vi "Build Start Stop Graph Legend.vi"() -> (2 "Stop Legend Graph":string, 3 "Start Legend Graph":string)   [LabVIEW 2021, in "TAF Proj Document Type.lvlib" / "TAF Proj.lvclass"]
uses:
  <vilib>/Wovalab/AntiDoc/Document Type/Add-ons/LabVIEW TAF Project/TAF Proj/TAF Proj.lvclass
  <vilib>/Wovalab/AntiDoc/GraphBuilder/Renderer/Graphviz/Graphviz.lvclass
  C:/Program Files (x86)/National Instruments/LabVIEW 2021/vi.lib/Wovalab/AntiDoc/GraphBuilder/Renderer/Renderer.lvclass
  <vilib>/Wovalab/AntiDoc/GraphBuilder/Shapes/Edge/Graphviz/Graphviz Edge Shape.lvclass
  <vilib>/Wovalab/AntiDoc/GraphBuilder/Shapes/Edge/Graphviz/Shape.ctl
  <vilib>/Wovalab/AntiDoc/GraphBuilder/Shapes/Edge/Graphviz/Colors.ctl
  <vilib>/Wovalab/AntiDoc/GraphBuilder/Shapes/Node/Graphviz/Colors.ctl
  <vilib>/Wovalab/AntiDoc/GraphBuilder/Shapes/Node/Graphviz/Shape.ctl
  <vilib>/Wovalab/AntiDoc/GraphBuilder/Renderer/Graphviz/Graph Direction.ctl
  <vilib>/Wovalab/AntiDoc/GraphBuilder/Renderer/Graphviz/Specific Edge Shape Def.ctl
  <vilib>/Wovalab/AntiDoc/GraphBuilder/Renderer/Graphviz/Specific Node Shape Def.ctl
  <vilib>/Wovalab/AntiDoc/GraphBuilder/Shapes/Node/Graphviz/Graphviz Node Shape.lvclass
  <vilib>/Wovalab/AntiDoc/GraphBuilder/Node/Node.lvclass
  <vilib>/Wovalab/AntiDoc/GraphBuilder/Graph/Graph.lvclass
  <vilib>/Wovalab/AntiDoc/GraphBuilder/Edge/Edge.lvclass
  <vilib>/Wovalab/AntiDoc/Document Type/Add-ons/LabVIEW TAF Project/TAF Proj Document Type.lvlib
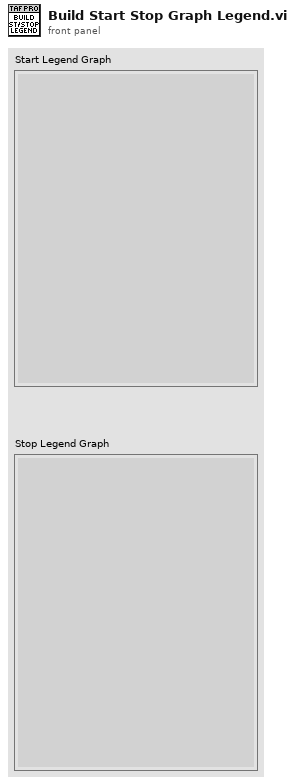
[diagram p1: front panel]
types:
  T1 = typedef "GraphBuilder.lvlib/Graphviz Edge Shape.lvclass/Shape.ctl" = enum16{"box", "lbox", "rbox", "obox", "olbox", "orbox", "crow", "lcrow", "rcrow", "diamond", "ldiamond", "rdiamond", "odiamond", "oldiamond", "ordiamond", "dot", "odot", "inv", "linv", "rinv", "oinv", "olinv", "orinv", "none", "normal", "lnormal", "rnormal", "onormal", "olnormal", "ornormal", "tee", "ltee", "rtee", "vee", "lvee", "rvee", "curve", "lcurve", "rcurve", "icurve", "licurve", "ricurve"}
  T2 = typedef "GraphBuilder.lvlib/Graphviz Edge Shape.lvclass/Style.ctl" = enum8{"filled", "invisible", "diagonals", "rounded", "dashed", "dotted", "solid", "bold"}
  T3 = typedef "GraphBuilder.lvlib/Graphviz Edge Shape.lvclass/Colors.ctl" = enum16{"aliceblue", "antiquewhite", "aqua", "aquamarine", "azure", "beige", "bisque", "black", "blanchedalmond", "blue", "blueviolet", "brown", "burlywood", "cadetblue", "chartreuse", "chocolate", "coral", "cornflowerblue", "cornsilk", "crimson", "cyan", "darkblue", "darkcyan", "darkgoldenrod", "darkgray", "darkgreen", "darkgrey", "darkkhaki", "darkmagenta", "darkolivegreen", "darkorange", "darkorchid", "darkred", "darksalmon", "darkseagreen", "darkslateblue", "darkslategray", "darkslategrey", "darkturquoise", "darkviolet", "deeppink", "deepskyblue", "dimgray", "dimgrey", "dodgerblue", "firebrick", "floralwhite", "forestgreen", "fuchsia", "gainsboro", "ghostwhite", "gold", "goldenrod", "gray", "green", "greenyellow", "grey", "honeydew", "hotpink", "indianred", "indigo", "ivory", "khaki", "lavender", "lavenderblush", "lawngreen", "lemonchiffon", "lightblue", "lightcoral", "lightcyan", "lightgoldenrodyellow", "lightgray", "lightgreen", "lightgrey", "lightpink", "lightsalmon", "lightseagreen", "lightskyblue", "lightslategray", "lightslategrey", "lightsteelblue", "lightyellow", "lime", "limegreen", "linen", "magenta", "maroon", "mediumaquamarine", "mediumblue", "mediumorchid", "mediumpurple", "mediumseagreen", "mediumslateblue", "mediumspringgreen", "mediumturquoise", "mediumvioletred", "midnightblue", "mintcream", "mistyrose", "moccasin", "navajowhite", "navy", "oldlace", "olive", "olivedrab", "orange", "orangered", "orchid", "palegoldenrod", "palegreen", "paleturquoise", "palevioletred", "papayawhip", "peachpuff", "peru", "pink", "plum", "powderblue", "purple", "red", "rosybrown", "royalblue", "saddlebrown", "salmon", "sandybrown", "seagreen", "seashell", "sienna", "silver", "skyblue", "slateblue", "slategray", "slategrey", "snow", "springgreen", "steelblue", "tan", "teal", "thistle", "tomato", "turquoise", "violet", "wheat", "white", "whitesmoke", "yellow", "yellowgreen"}
  T4 = typedef "GraphBuilder.lvlib/Graphviz Node Shape.lvclass/Colors.ctl" = enum16{"aliceblue", "antiquewhite", "aqua", "aquamarine", "azure", "beige", "bisque", "black", "blanchedalmond", "blue", "blueviolet", "brown", "burlywood", "cadetblue", "chartreuse", "chocolate", "coral", "cornflowerblue", "cornsilk", "crimson", "cyan", "darkblue", "darkcyan", "darkgoldenrod", "darkgray", "darkgreen", "darkgrey", "darkkhaki", "darkmagenta", "darkolivegreen", "darkorange", "darkorchid", "darkred", "darksalmon", "darkseagreen", "darkslateblue", "darkslategray", "darkslategrey", "darkturquoise", "darkviolet", "deeppink", "deepskyblue", "dimgray", "dimgrey", "dodgerblue", "firebrick", "floralwhite", "forestgreen", "fuchsia", "gainsboro", "ghostwhite", "gold", "goldenrod", "gray", "green", "greenyellow", "grey", "honeydew", "hotpink", "indianred", "indigo", "ivory", "khaki", "lavender", "lavenderblush", "lawngreen", "lemonchiffon", "lightblue", "lightcoral", "lightcyan", "lightgoldenrodyellow", "lightgray", "lightgreen", "lightgrey", "lightpink", "lightsalmon", "lightseagreen", "lightskyblue", "lightslategray", "lightslategrey", "lightsteelblue", "lightyellow", "lime", "limegreen", "linen", "magenta", "maroon", "mediumaquamarine", "mediumblue", "mediumorchid", "mediumpurple", "mediumseagreen", "mediumslateblue", "mediumspringgreen", "mediumturquoise", "mediumvioletred", "midnightblue", "mintcream", "mistyrose", "moccasin", "navajowhite", "navy", "oldlace", "olive", "olivedrab", "orange", "orangered", "orchid", "palegoldenrod", "palegreen", "paleturquoise", "palevioletred", "papayawhip", "peachpuff", "peru", "pink", "plum", "powderblue", "purple", "red", "rosybrown", "royalblue", "saddlebrown", "salmon", "sandybrown", "seagreen", "seashell", "sienna", "silver", "skyblue", "slateblue", "slategray", "slategrey", "snow", "springgreen", "steelblue", "tan", "teal", "thistle", "tomato", "turquoise", "violet", "wheat", "white", "whitesmoke", "yellow", "yellowgreen"}
  T5 = typedef "GraphBuilder.lvlib/Graphviz Node Shape.lvclass/Shape.ctl" = enum16{"box", "polygon", "ellipse", "oval", "circle", "point", "egg", "triangle", "plaintext", "plain", "diamond", "trapezium", "parallelogram", "house", "pentagon", "hexagon", "septagon", "octagon", "doublecircle", "doubleoctagon", "tripleoctagon", "invtriangle", "invtrapezium", "invhouse", "Mdiamond", "Msquare", "Mcircle", "rect", "rectangle", "square", "star", "none", "underline", "cylinder", "note", "tab", "folder", "box3D", "component", "promoter", "cds", "terminator", "utr", "primersite", "restrictionsite", "fivepoverhang", "threepoverhang", "noverhang", "assembly", "signature", "insulator", "ribosite", "rnastab", "proteasesite", "proteinstab", "rpromoter", "rarrow", "larrow", "lpromoter"}
  T6 = typedef "GraphBuilder.lvlib/Graphviz.lvclass/Specific Node Shape Def.ctl" = cluster{"Node ID":string, "Graphviz Node Shape":refnum<class "Graphviz Node Shape.lvclass">}
  T7 = typedef "GraphBuilder.lvlib/Graphviz.lvclass/Specific Edge Shape Def.ctl" = cluster{"Source Node ID":string, "Target Node ID":string, "Caption":string, "Graphviz Edge Shape":refnum<class "Graphviz Edge Shape.lvclass">}
  T8 = typedef "GraphBuilder.lvlib/Graphviz.lvclass/Graph Direction.ctl" = enum16{"Top to Bottom", "Left To Right", "Bottom to Top", "Right to Left"}
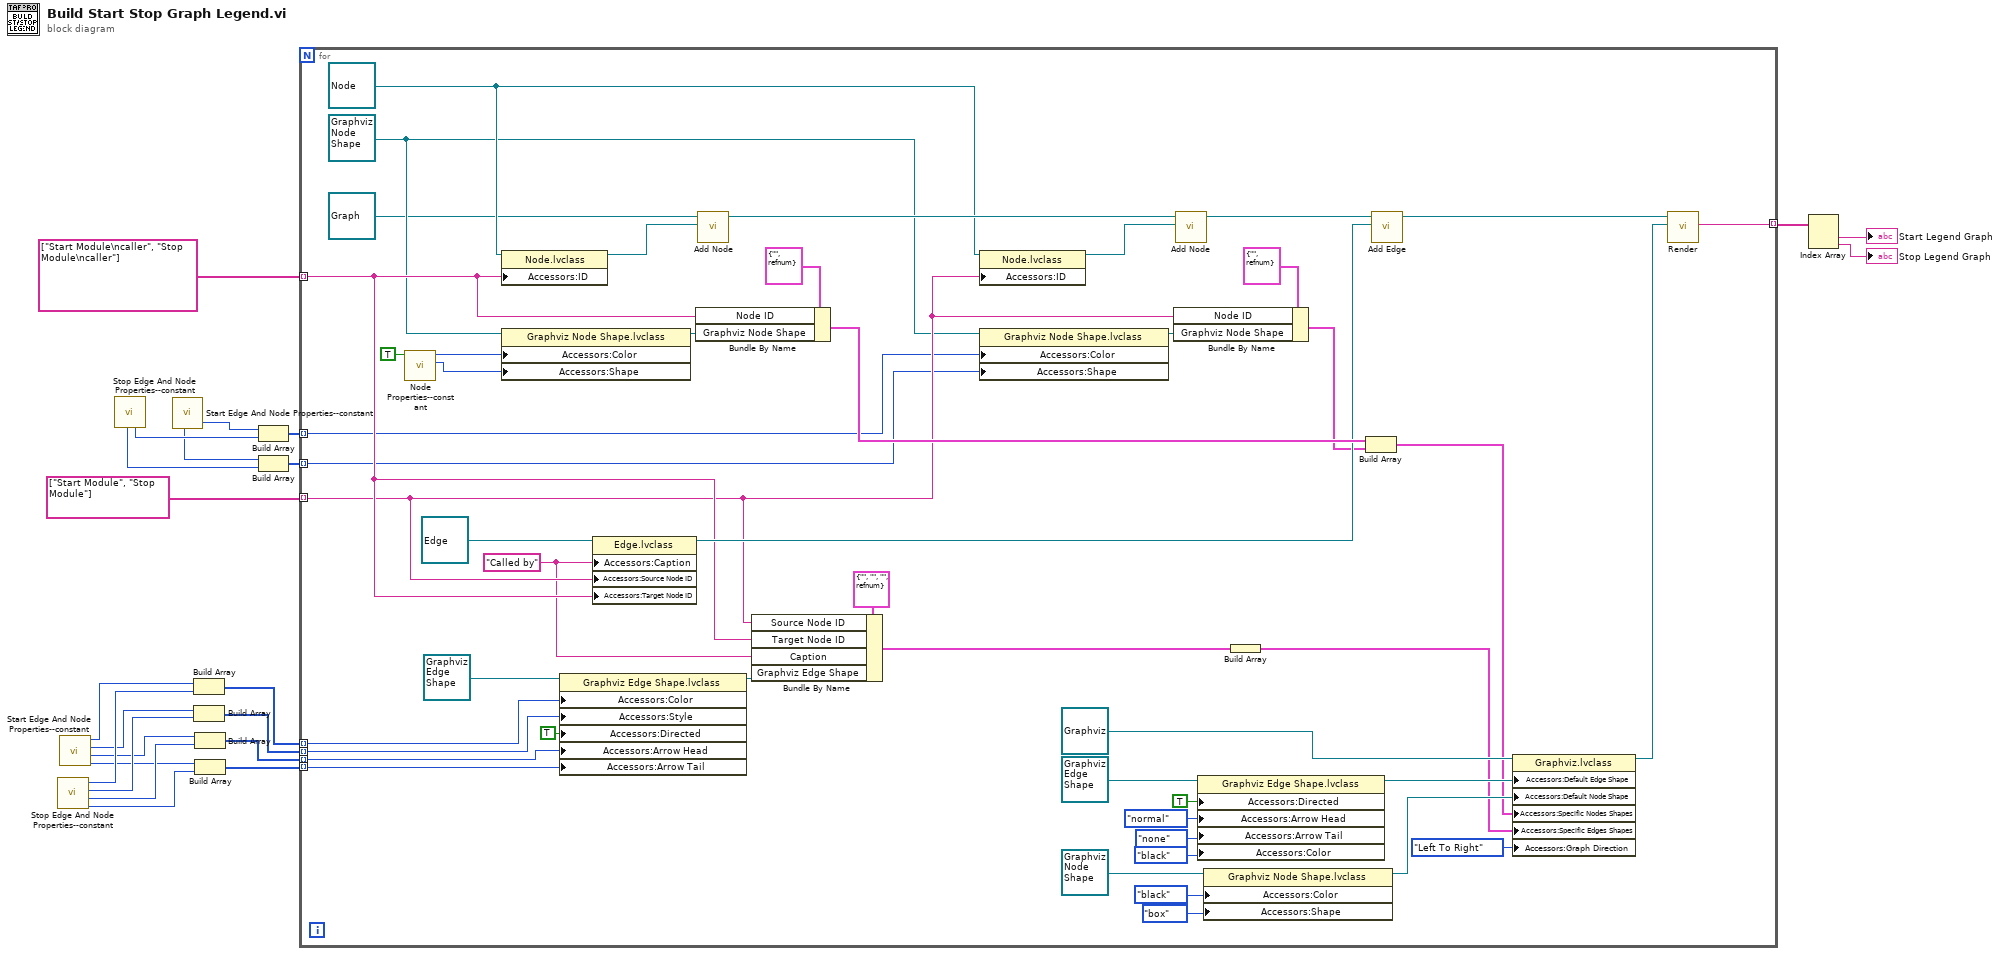
[diagram p0: block diagram]
diagram:
  n1 = call <vilib>:"Stop Edge And Node Properties--constant.vi"() -> ("Edge Arrow Tail"=w12:T1, "Edge Arrow Head"=w13:T1, "Edge Style"=w14:T2, "Edge Color"=w15:T3)  [unwired: 6 in, 2 out]
  n2 = call <vilib>:"Start Edge And Node Properties--constant.vi"() -> ("Edge Arrow Tail"=w5:T1, "Edge Arrow Head"=w7:T1, "Edge Style"=w9:T2, "Edge Color"=w11:T3)  [unwired: 6 in, 2 out]
  n3 = call <vilib>:"Stop Edge And Node Properties--constant.vi"() -> ("Node Color"=w20:T4, "Node Shape"=w18:T5)  [unwired: 6 in, 4 out]
  n4 = call <vilib>:"Start Edge And Node Properties--constant.vi"() -> ("Node Color"=w21:T4, "Node Shape"=w19:T5)  [unwired: 6 in, 4 out]
  n5 = Build Array(w11, w15) -> (w10:T3[])
  n6 = Build Array(w9, w14) -> (w8:T2[])
  n7 = Build Array(w7, w13) -> (w6:T1[])
  n8 = Build Array(w5, w12) -> (w4:T1[])
  n9 = Build Array(w21, w20) -> (w17:T4[])
  n10 = Build Array(w19, w18) -> (w16:T5[])
  n11 = for {
    tunnel: [w54] -> w3 mode=indexing
    tunnel: string[] ["Start Module\ncaller", "Stop Module\ncaller"] -> [w47] mode=indexing
    tunnel: w10 -> [w46] mode=indexing
    tunnel: w8 -> [w45] mode=indexing
    tunnel: w6 -> [w44] mode=indexing
    tunnel: w4 -> [w43] mode=indexing
    tunnel: string[] ["Start Module", "Stop Module"] -> [w38] mode=indexing
    tunnel: w17 -> [w34] mode=indexing
    tunnel: w16 -> [w33] mode=indexing
    w24 = "Called by" ("Caption")
    w28 = refnum<class "Graphviz Node Shape.lvclass"> refnum ("GraphBuilder.lvlib:Graphviz Node Shape.lvclass")
    w29 = refnum<class "Node.lvclass"> refnum ("GraphBuilder.lvlib:Node.lvclass")
    n12 = call <vilib>:"Node Properties--constant.vi"("Lvlib"=TRUE) -> ("Shape"=w49:T5, "Color"=w50:T4)  [unwired: 9 in]
    n13 = property class="Node.lvclass"(reference=w29, "Accessors:ID"=w47) -> (reference out=w30:refnum<class "Node.lvclass">)  [unwired: 1 in, 1 out]
    n14 = property class="Graphviz Node Shape.lvclass"(reference=w28, "Accessors:Color"=w50, "Accessors:Shape"=w49) -> (reference out=w32:refnum<class "Graphviz Node Shape.lvclass">)  [unwired: 1 in, 1 out]
    n15 = property class="Graphviz Edge Shape.lvclass"(reference=refnum<class "Graphviz Edge Shape.lvclass"> refnum ("Graphviz Edge Shape"), "Accessors:Color"=w46, "Accessors:Style"=w45, "Accessors:Directed"=TRUE ("Directed"), "Accessors:Arrow Head"=w44, "Accessors:Arrow Tail"=w43) -> (reference out=w59:refnum<class "Graphviz Edge Shape.lvclass">)  [unwired: 1 in, 1 out]
    n16 = property class="Edge.lvclass"(reference=refnum<class "Edge.lvclass"> refnum ("Edge"), "Accessors:Caption"=w24, "Accessors:Source Node ID"=w38, "Accessors:Target Node ID"=w47) -> (reference out=w51:refnum<class "Edge.lvclass">)  [unwired: 1 in, 1 out]
    n17 = Bundle By Name(cluster=T6 {"Node ID"="", "Graphviz Node Shape"=refnum} ("Specific Node Shape"), "Node ID"=w47, "Graphviz Node Shape"=w32) -> (w53:T6)
    n18 = call-dynamic "Add Node.vi"("Node"=w30, "Graph in"=refnum<class "Graph.lvclass"> refnum ("GraphBuilder.lvlib:Graph.lvclass")) -> ("Graph out"=w42:refnum<class "Graph.lvclass">)  [unwired: 8 in, 1 out]
    n19 = Bundle By Name(cluster=T7 {"Source Node ID"="", "Target Node ID"="", "Caption"="", "Graphviz Edge Shape"=refnum} ("Specific Edge Shape"), "Source Node ID"=w38, "Target Node ID"=w47, "Caption"=w24, "Graphviz Edge Shape"=w59) -> (w57:T7)
    n20 = property class="Node.lvclass"(reference=w29, "Accessors:ID"=w38) -> (reference out=w35:refnum<class "Node.lvclass">)  [unwired: 1 in, 1 out]
    n21 = property class="Graphviz Node Shape.lvclass"(reference=w28, "Accessors:Color"=w34, "Accessors:Shape"=w33) -> (reference out=w37:refnum<class "Graphviz Node Shape.lvclass">)  [unwired: 1 in, 1 out]
    n22 = Bundle By Name(cluster=T6 {"Node ID"="", "Graphviz Node Shape"=refnum} ("Specific Node Shape"), "Node ID"=w38, "Graphviz Node Shape"=w37) -> (w39:T6)
    n23 = call-dynamic "Add Node.vi"("Node"=w35, "Graph in"=w42) -> ("Graph out"=w41:refnum<class "Graph.lvclass">)  [unwired: 8 in, 1 out]
    n24 = property class="Graphviz Edge Shape.lvclass"(reference=refnum<class "Graphviz Edge Shape.lvclass"> refnum ("GraphBuilder.lvlib:Graphviz Edge Shape.lvclass"), "Accessors:Directed"=TRUE ("Directed"), "Accessors:Arrow Head"=Shape."normal" ("Arrow Head"), "Accessors:Arrow Tail"=Shape."none" ("Arrow Tail"), "Accessors:Color"=Colors."black" ("Color")) -> (reference out=w70:refnum<class "Graphviz Edge Shape.lvclass">)  [unwired: 1 in, 1 out]
    n25 = property class="Graphviz Node Shape.lvclass"(reference=refnum<class "Graphviz Node Shape.lvclass"> refnum ("GraphBuilder.lvlib:Graphviz Node Shape.lvclass"), "Accessors:Color"=Colors."black" ("Color"), "Accessors:Shape"=Shape."box" ("Shape")) -> (reference out=w71:refnum<class "Graphviz Node Shape.lvclass">)  [unwired: 1 in, 1 out]
    n26 = Build Array(w57) -> (w56:T7[])
    n27 = Build Array(w53, w39) -> (w40:T6[])
    n28 = call-dynamic "Add Edge.vi"("Edge"=w51, "Graph in"=w41) -> ("Graph out"=w52:refnum<class "Graph.lvclass">)  [unwired: 8 in, 1 out]
    n29 = property class="Graphviz.lvclass"(reference=refnum<class "Graphviz.lvclass"> refnum ("GraphBuilder.lvlib:Graphviz.lvclass"), "Accessors:Default Edge Shape"=w70, "Accessors:Default Node Shape"=w71, "Accessors:Specific Nodes Shapes"=w40, "Accessors:Specific Edges Shapes"=w56, "Accessors:Graph Direction"=Graph_Direction."Left To Right" ("Graph Direction")) -> (reference out=w72:refnum<class "Graphviz.lvclass">)  [unwired: 1 in, 1 out]
    n30 = call-dynamic "Render.vi"("Renderer"=w72, "Graph in"=w52) -> ("Rendered Stream"=w54:string)  [unwired: 7 in, 2 out]
  }
  n31 = Index Array(array=w3) -> (element #1=→"Start Legend Graph":string, element #2=→"Stop Legend Graph":string)  [unwired: 2 in]
